vi "Add Rx Monitor Section and Status and Logging.vi"(8 "error in":errorcluster, 10 "session_rx_monitor":T1={"DefaultCronoMode"=1, "GlbMonBufferSizeIn"=0, "CaptureMode"=0, "MaxFileSizeMB"=1, "Strobe"=0, "TriggerPosition"=0} {"Strobe" items=["FDX_MON_STROBE_DIS", "FDX_MON_STROBE_STOP", "FDX_MON_STROBE_START"]; "CaptureMode" items=["FDX_MON_SINGLE ", "FDX_MON_CONTINUOUS", "FDX_MON_SELECTIVE", "FDX_MON_RECORDING", "FDX_MON_REROS", "FDX_MON_HMU"]; "DefaultCronoMode" items=["FDX_RX_DEFAULT_ENA_CNT", "FDX_RX_DEFAULT_MON_ENA_ALL", "FDX_RX_DEFAULT_MON_ENA_GOOD"]}, 11 "port ref":T2 format="%.0x") -> (0 "error out":errorcluster, 3 "port ref out":T2 format="%.0x")   [LabVIEW 2020, in "AIM ARINC 664 Scripting.lvlib"]
doc: "Add an Rx Monitor based on the configuration input."
uses:
  AIM ARINC 664 Scripting.lvlib
  <vilib>/Utility/SystemLogging/NI_SystemLogging.lvlib
  <vilib>/NI VeriStand/Custom Device API/Custom Device Item Ref.ctl
  <vilib>/NI VeriStand/Custom Device API/Custom Device API.lvlib
  Import/_typedefs/session_rx_monitor.ctl
  Import/AIM ARINC 664 Import.lvlib
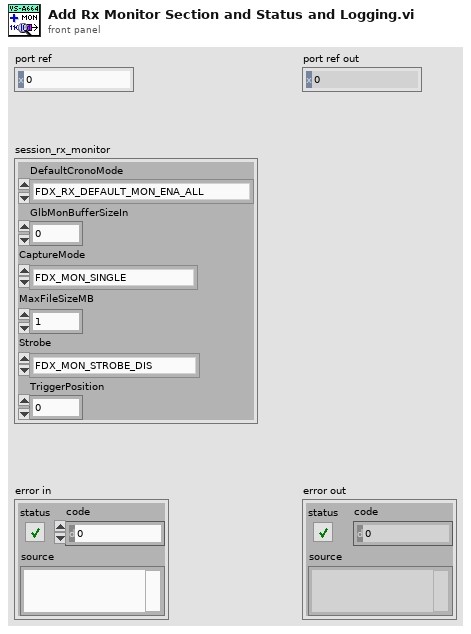
[diagram p1: front panel]
types:
  T1 = typedef "AIM ARINC 664 Import.lvlib/session_rx_monitor.ctl" = cluster{"DefaultCronoMode":u32, "GlbMonBufferSizeIn":u32, "CaptureMode":u32, "MaxFileSizeMB":u32, "Strobe":u32, "TriggerPosition":u32}
  T2 = typedef "Custom Device API.lvlib/Custom Device Item Ref.ctl" = u64
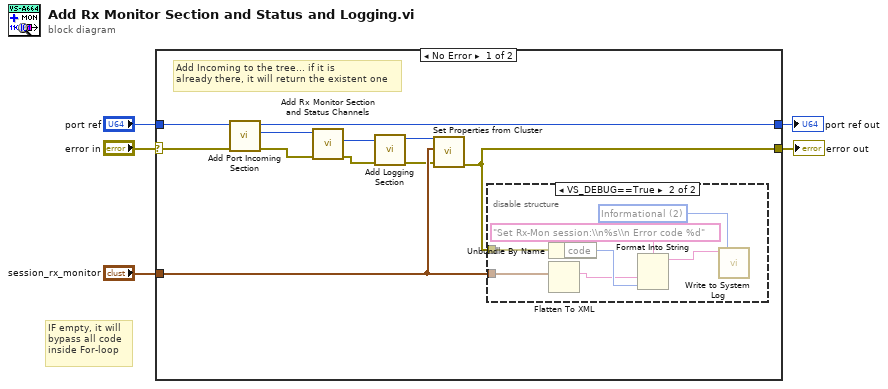
[diagram p0: block diagram]
diagram:
  # "IF empty, it will\nbypass all code \ninside For-loop"
  n1 = case shown="No Error" "error in" {
    selector: "error in" -> [w6 w25]
    tunnel: "port ref" -> [w16 w24]
    tunnel: [w15 w25] -> w4
    tunnel: [w14 w24] -> w3
    tunnel: "session_rx_monitor" -> [w13 _]
    frame No Error {
      # "Add Incoming to the tree... if it is \nalready there, it will return the existent one"
      n2 = call "Add Port Incoming Section.vi"("error in"=w6, "ports ref"=w16) -> ("error out"=w12:errorcluster, "incoming section ref out"=w11:T2, "ports ref out"=w14:T2)  [unwired: 7 in]
      n3 = call "Add Rx Monitor Section and Status Channels.vi"("error in"=w12, "port ref in"=w11) -> ("error out"=w9:errorcluster, "Rx monitor ref out"=w10:T2)  [unwired: 6 in, 2 out]
      n4 = call "Add Logging Section.vi"("error in"=w9, "custom device ref"=w10) -> ("error out"=w8:errorcluster, "custom device ref out"=w7:T2)  [unwired: 6 in, 2 out]
      n5 = call "Set Properties from Cluster.vi"("error in"=w8, "Variant Cluster"=w13, "item ref in"=w7) -> ("error out"=w15:errorcluster)  [unwired: 7 in, 1 out]
      n6 = disable-structure shown="VS_DEBUG==True" {
        disable-tunnel: w15 -> [_ w19]
        disable-tunnel: w13 -> [_ w18]
        frame condition #0 (active) {
        }
        frame condition #1 {
          w21 = 2 items=["Error", "Warning", "Informational"] ("severity")
          n7 = Unbundle By Name(w19) -> ("code"=w20:i32)
          n8 = Flatten To XML(6:w18) -> (2:w17:string)
          n9 = Format Into String(format string="Set Rx-Mon session:\\n%s\\n Error code %d", w17, w20) -> (resulting string=w22:string)  [unwired: 2 in, 1 out]
          n10 = call <vilib>:"Write to System Log.vi"("severity"=w21, "message"=w22) -> ()  [unwired: 9 in, 1 out]
        }
      }
    }
    frame Error {
    }
  }
  "error out" <- w4
  "port ref out" <- w3
